vi "pressure_change.vi"(1 "Pressure Voltage (V)":dynamicdata(graph)) -> (0 "Streamwise dP (kPa)":dbl)   [LabVIEW 2015]
uses:
  <vilib>/express/express shared/transition.llb/Dynamic To Waveform Array.vi
  <vilib>/express/express arith-compare/Formula/Block/exnFormulaBlock how many pts in the wave.vi
  <vilib>/express/express shared/ex_Modify Signal Name.vi
  <vilib>/express/express shared/transition.llb/Waveform Array To Dynamic.vi
  <vilib>/express/express arith-compare/Formula/XNode/ExpressFormulaBlockNode.xnode
panel:
  in  "Pressure Voltage (V)":dbl
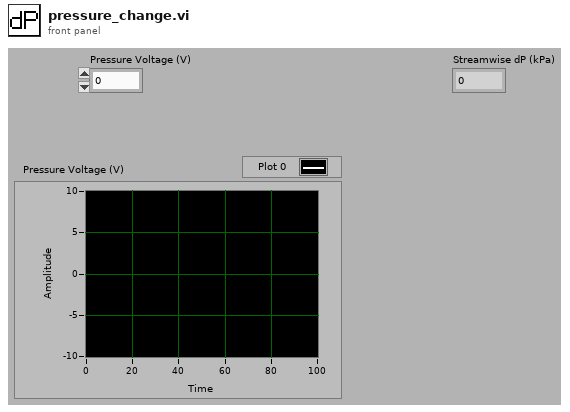
[diagram p1: front panel]
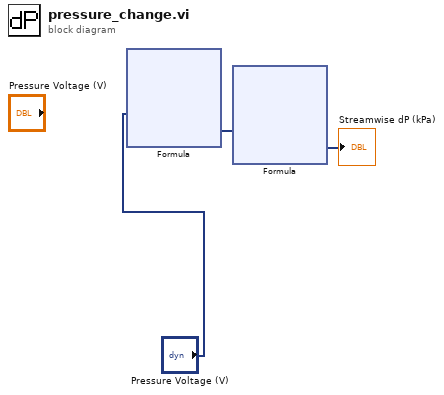
[diagram p0: block diagram]
diagram:
  n1 = xnode "Formula"("I"="Pressure Voltage (V)") -> ("Result"=w3:dynamicdata)  [unwired: 1 in, 1 out]
  n2 = xnode "Formula"("P"=w3) -> ("Result"=→"Streamwise dP (kPa)":dynamicdata)  [unwired: 1 in, 1 out]
